vi "Find All Paths_DFS.vi"(8 "error in (no error)":errorcluster, 9 "End Vertex":i32=9999, 10 "Start Vertex":i32=1111, 11 "Graph Variant":variant) -> (0 "error out":errorcluster, 3 "Paths DFS":i32[][](array[numeric]))   [LabVIEW 2013, in "Graph.lvclass"]
uses:
  Graph.lvclass
  Controls/StackDataType.ctl
  <userlib>/_OpenG.lib/array/array.llb/Filter 1D Array (I32)__ogtk.vi
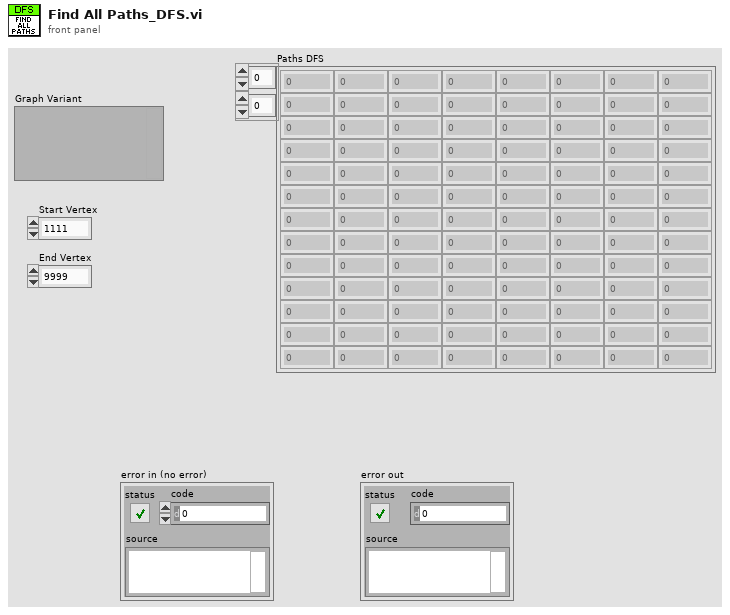
[diagram p1: front panel]
types:
  T1 = typedef "Graph.lvclass/StackDataType.ctl" = cluster{"Vertex":i32, "Path":i32[]}
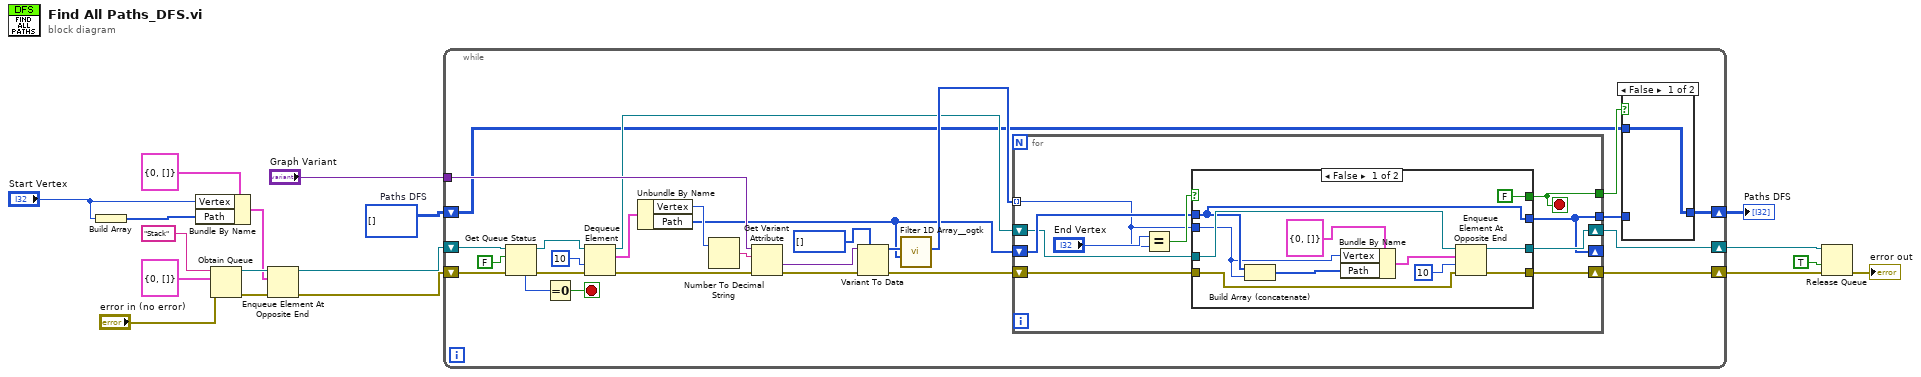
[diagram p0: block diagram]
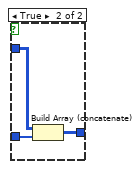
[diagram p2: hidden frame]
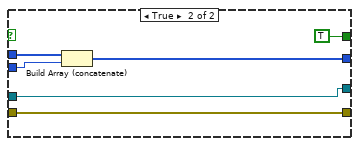
[diagram p3: hidden frame]
diagram:
  w5 = i32[][] []  # Paths DFS
  n1 = Build Array("Start Vertex") -> (w11:i32[])
  n2 = Bundle By Name(cluster=T1 {"Vertex"=0, "Path"=[]} ("element"), "Vertex"="Start Vertex", "Path"=w11) -> (w10:T1)
  n3 = Obtain Queue(name (unnamed)="Stack", element data type=T1 {"Vertex"=0, "Path"=[]}, error in (no error)="error in (no error)") -> (queue out=w15:refnum<queue>, error out=w14:errorcluster)  [unwired: 2 in, 1 out]
  n4 = Enqueue Element At Opposite End(queue=w15, element=w10, error in (no error)=w14) -> (queue out=w9:refnum<queue>, error out=w8:errorcluster)  [unwired: 1 in, 1 out]
  n5 = while {
    shift-right: [w25] -> w6
    shift-left: w9 -> [w44]
    shift-right: [w26] -> w7
    shift-left: w8 -> [w45]
    tunnel: "Graph Variant" -> [w39]
    shift-right: [w19] -> w4
    shift-left: w5 -> [w20]
    stop <- w42 stop-if-true
    n6 = Get Queue Status(queue=w44, return elements? (F)=FALSE, error in (no error)=w45) -> (queue out=w40:refnum<queue>, error out=w41:errorcluster, # elements in queue=w43:i32)  [unwired: 5 out]
    n7 = Equal To 0?(x=w43) -> (x = 0?=w42:bool)
    n8 = Dequeue Element(queue=w40, timeout in ms (-1)=10, error in (no error)=w41) -> (queue out=w28:refnum<queue>, element=w37:T1, error out=w38:errorcluster)  [unwired: 1 out]
    n9 = Unbundle By Name(w37) -> ("Vertex"=w36:i32, "Path"=w29:i32[])
    n10 = Number To Decimal String(number=w36) -> (decimal integer string=w35:string)  [unwired: 1 in]
    n11 = Get Variant Attribute(Variant=w39, name=w35, error in=w38) -> (value=w33:variant, error out=w34:errorcluster)  [unwired: 1 in, 2 out]
    n12 = Variant To Data(error in=w34, type=i32[] [], Variant=w33) -> (data=w31:i32[], error out=w27:errorcluster)
    n13 = call-poly <userlib>:"Filter 1D Array__ogtk.vi"("items to filter"=w29, "array"=w31) -> ("filtered array"=w30:i32[])  [unwired: 4 in, 1 out]
    n14 = for {
      tunnel: w30 -> [w56] mode=indexing
      shift-right: [w51] -> _
      shift-left: w29 -> [w57]
      shift-right: [w54] -> w25
      shift-left: w28 -> [w55]
      shift-right: [w52] -> w26
      shift-left: w27 -> [w53]
      tunnel: [w51] -> w21
      tunnel: [w50] -> w22
      stop <- w50 stop-if-true
      n15 = Equal?(x="End Vertex", y=w56) -> (x = y?=w58:bool)
      n16 = case shown="False" w58 {
        tunnel: [FALSE TRUE] -> w50
        tunnel: w57 -> [w64 w75]
        tunnel: w56 -> [w63 w74]
        tunnel: [w64 w73] -> w51
        tunnel: w55 -> [w69 w72]
        tunnel: [w68 w72] -> w54
        tunnel: w53 -> [w67 w71]
        tunnel: [w66 w71] -> w52
        frame False {
          n17 = Build Array (concatenate)(w64, w63) -> (w62:i32[])
          n18 = Bundle By Name(cluster=T1 {"Vertex"=0, "Path"=[]} ("element"), "Vertex"=w63, "Path"=w62) -> (w61:T1)
          n19 = Enqueue Element At Opposite End(queue=w69, element=w61, timeout in ms (-1)=10, error in (no error)=w67) -> (queue out=w68:refnum<queue>, error out=w66:errorcluster)  [unwired: 1 out]
        }
        frame True {
          n20 = Build Array (concatenate)(w75, w74) -> (w73:i32[])
        }
      }
    }
    n21 = case shown="False" w22 {
      tunnel: w21 -> [_ w48]
      tunnel: w20 -> [w46 w49]
      tunnel: [w46 w47] -> w19
      frame False {
      }
      frame True {
        n22 = Build Array (concatenate)(w49, w48) -> (w47:i32[][])
      }
    }
  }
  "Paths DFS" <- w4
  n23 = Release Queue(queue=w6, force destroy? (F)=TRUE, error in (no error)=w7) -> (error out=→"error out":errorcluster)  [unwired: 2 out]
